vi "Error.vi"(8 "error in (no error)":errorcluster, 11 "Modulo a obtener":T1=enum."Error") -> (0 "error out":errorcluster)   [LabVIEW 2018]
uses:
  Comunes/Controles/Lista Modulos.ctl
  Comunes/Controles/FGV Opciones.ctl
  Comunes/Comunicacion/Mensajes.lvlib
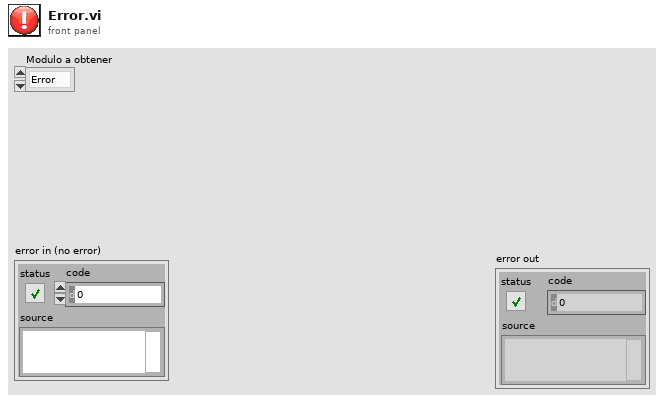
[diagram p1: front panel]
types:
  T1 = typedef "Lista Modulos.ctl" = enum16{"Math", "Error", "Front", "Database", "Nuevos items"}
  T2 = typedef "FGV Opciones.ctl" = enum16{"Get", "Create", "Destroy"}
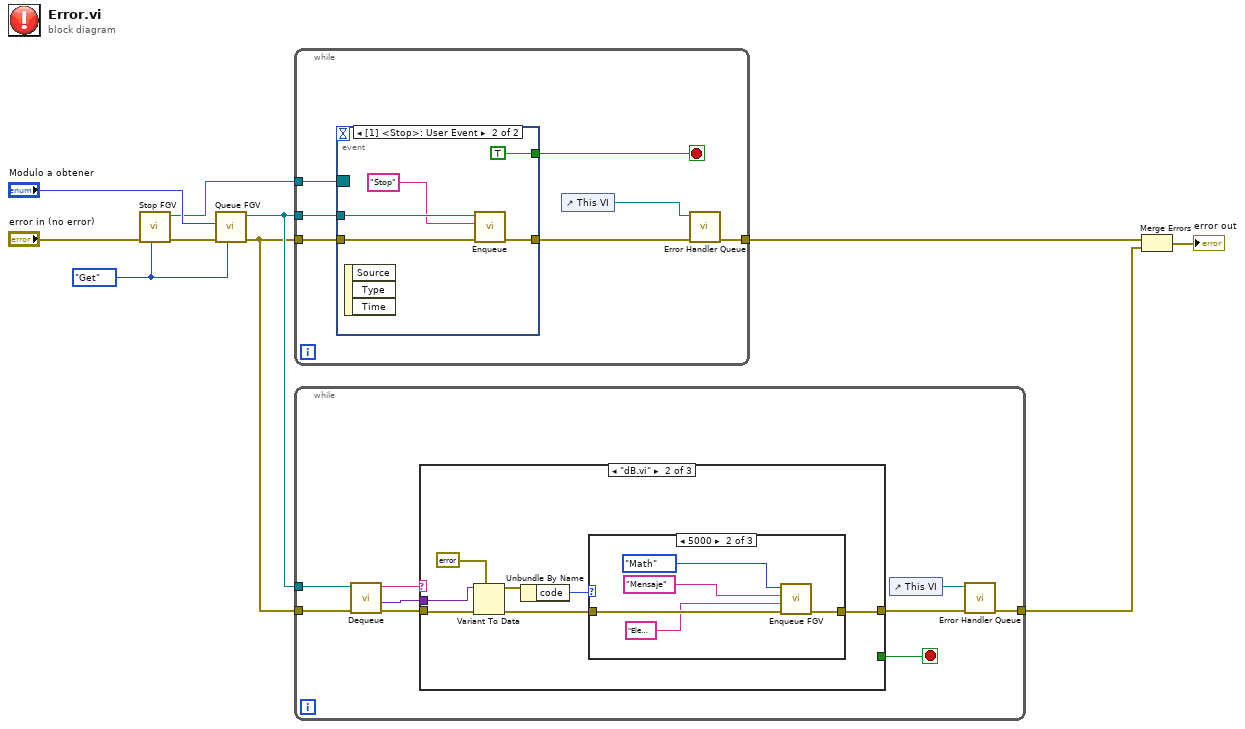
[diagram p0: block diagram]
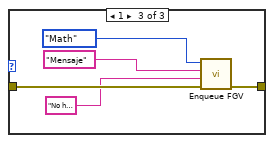
[diagram p4: hidden frame]
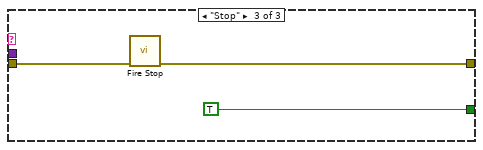
[diagram p5: hidden frame]
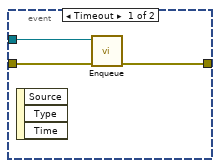
[diagram p6: hidden frame]
diagram:
  w1 = FGV_Opciones."Get" ("Enum")
  n1 = call "Stop FGV.vi"("Enum"=w1, "error in (no error)"="error in (no error)") -> ("error out"=w2:errorcluster, "Event Registration Refnum"=w4:refnum<event-registration>)  [unwired: 7 in, 1 out]
  n2 = call "Queue FGV.vi"("Enum"=w1, "error in (no error)"=w2, "Modulo a obtener"="Modulo a obtener") -> ("error out"=w8:errorcluster, "Queue Ref"=w9:refnum<queue>)  [unwired: 7 in]
  n3 = while {
    tunnel: w9 -> [w17]
    tunnel: w8 -> [w16]
    tunnel: [w14] -> w7
    tunnel: w4 -> [w12]
    stop <- w11 stop-if-true
    n4 = event shown="[1] <Stop>: User Event" {
      selector: w12 -> [_ _]
      dyn-events: _ -> [_ _]
      timeout: _ -> [_ _]
      tunnel: w17 -> [w20 w23]
      tunnel: w16 -> [w19 w24]
      tunnel: [w18 w21] -> w13
      tunnel: [_ TRUE] -> w11
      event Timeout {
        n5 = event-data() -> ()  [unwired: 1 in, 3 out]
        n6 = call "Enqueue.vi"("error in (no error)"=w19, "Queue in"=w20) -> ("error out"=w18:errorcluster)  [unwired: 9 in]
      }
      event User Event {
        n7 = event-data() -> ()  [unwired: 1 in, 3 out]
        n8 = call "Enqueue.vi"("error in (no error)"=w24, "Mensaje"="Stop", "Queue in"=w23) -> ("error out"=w21:errorcluster)  [unwired: 8 in]
      }
    }
    n9 = control-ref of="This VI"() -> (w15:refnum<vi>)
    n10 = call "Error Handler Queue.vi"("error in (no error)"=w13, "VI Refnum"=w15) -> ("error out"=w14:errorcluster)  [unwired: 9 in]
  }
  n11 = while {
    tunnel: w9 -> [w34]
    tunnel: w8 -> [w33]
    tunnel: [w27] -> w6
    stop <- w26 stop-if-true
    n12 = call "Dequeue.vi"("error in (no error)"=w33, "Queue in"=w34) -> ("error out"=w29:errorcluster, "Dato"=w31:variant, "Mensaje"=w32:string)  [unwired: 7 in]
    n13 = case shown="\"dB.vi\"" w32 {
      tunnel: w31 -> [_ w41 _]
      tunnel: w29 -> [w35 w42 w56]
      tunnel: [w35 w38 w54] -> w28
      tunnel: [_ _ TRUE] -> w26
      frame "False", Default {
      }
      frame "dB.vi" {
        n14 = Variant To Data(error in=w42, type=errorcluster {"status"=FALSE, "code"=0, "source"=""} ("error in (no error)"), Variant=w41) -> (data=w37:errorcluster, error out=w39:errorcluster)
        n15 = Unbundle By Name(w37) -> ("code"=w36:i32)
        n16 = case shown="5000" w36 {
          tunnel: w39 -> [w43 w48 w53]
          tunnel: [w43 w47 w52] -> w38
          frame 0, Default {
          }
          frame 5000 {
            n17 = call "Enqueue FGV.vi"("error in (no error)"=w48, "Dato"="Elemento ya existente" ("Mensaje"), "Mensaje"="Mensaje", "Modulo a obtener"=Lista_Modulos."Math") -> ("error out"=w47:errorcluster)  [unwired: 7 in]
          }
          frame 1 {
            n18 = call "Enqueue FGV.vi"("error in (no error)"=w53, "Dato"="No hay conexxion a tinternet" ("Mensaje"), "Mensaje"="Mensaje", "Modulo a obtener"=Lista_Modulos."Math") -> ("error out"=w52:errorcluster)  [unwired: 7 in]
          }
        }
      }
      frame "Stop" {
        n19 = call "Fire Stop.vi"("error in (no error)"=w56) -> ("error out"=w54:errorcluster)  [unwired: 10 in]
      }
    }
    n20 = control-ref of="This VI"() -> (w30:refnum<vi>)
    n21 = call "Error Handler Queue.vi"("error in (no error)"=w28, "VI Refnum"=w30) -> ("error out"=w27:errorcluster)  [unwired: 9 in]
  }
  n22 = Merge Errors(w7, w6) -> (→"error out":errorcluster)
